vi "calculate.vi"(8 "error in (no error)":errorcluster, 10 "Numbers.lvclass":refnum<class "Numbers.lvclass">, 11 "Add in":refnum<class "Add.lvclass">) -> (0 "error out":errorcluster, 3 "Add out":refnum<class "Add.lvclass">)   [LabVIEW 2017, in "Add.lvclass"]
uses:
  Add.lvclass
  Numbers Class/Numbers.lvclass
  Numbers Class/Numbers.lvclass/Numbers.ctl
  Add.lvclass/Add.ctl
  Chain Class/Chain.lvclass
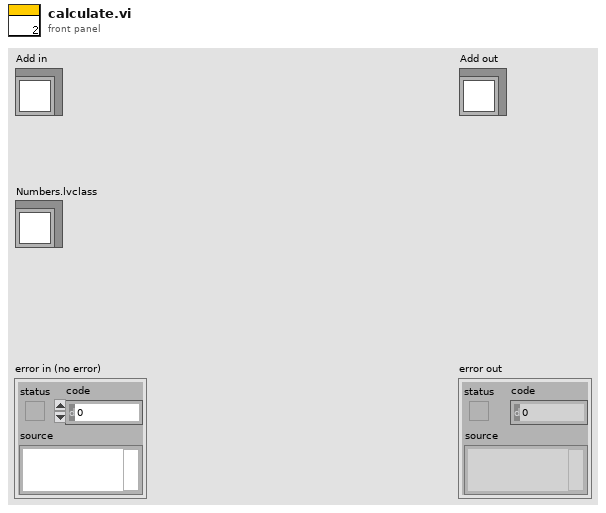
[diagram p1: front panel]
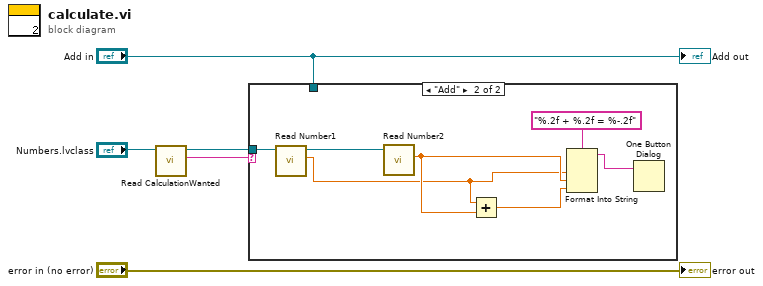
[diagram p0: block diagram]
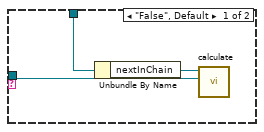
[diagram p2: hidden frame]
diagram:
  n1 = call "Read CalculationWanted.vi"("Numbers in"="Numbers.lvclass") -> ("CalculationWanted"=w3:string, "Numbers out"=w2:refnum<class "Numbers.lvclass">)  [unwired: 8 in, 1 out]
  n2 = case shown="\"Add\"" w3 {
    tunnel: w2 -> [w8 w15]
    tunnel: "Add in" -> [w7 _]
    frame "False", Default {
      n3 = Unbundle By Name(w7) -> ("nextInChain"=w6:refnum<class "Chain.lvclass">)
      n4 = call-dynamic "calculate.vi"("Numbers.lvclass"=w8, "Chain in"=w6) -> ()  [unwired: 8 in, 2 out]
    }
    frame "Add" {
      n5 = call "Read Number1.vi"("Numbers in"=w15) -> ("Number1"=w9:dbl, "Numbers out"=w14:refnum<class "Numbers.lvclass">)  [unwired: 8 in, 1 out]
      n6 = call "Read Number2.vi"("Numbers in"=w14) -> ("Number2"=w10:dbl)  [unwired: 8 in, 2 out]
      n7 = Add(x=w9, y=w10) -> (x+y=w12:dbl)
      n8 = Format Into String(format string="%.2f + %.2f = %-.2f", w9, w10, w12) -> (resulting string=w11:string)  [unwired: 2 in, 1 out]
      n9 = One Button Dialog(message=w11) -> ()  [unwired: 1 in, 1 out]
    }
  }
  "error out" <- "error in (no error)"
  "Add out" <- "Add in"
